vi "TestInsertIntoPanel_OK.vi"(8 "error in (no error)":errorcluster, 11 "TestCase in":refnum<class "TestProtectedSubpanel.lvclass">) -> (0 "error out":errorcluster, 3 "TestCase out":refnum<class "TestProtectedSubpanel.lvclass">)   [LabVIEW 2015, in "TestProtectedSubpanel.lvclass"]
uses:
  TestProtectedSubpanel.lvclass
  TestProtectedSubpanel.lvclass/TestProtectedSubpanel.ctl
  Framework/IViewable/ProtectedSubpanel/ProtectedSubpanel.lvclass
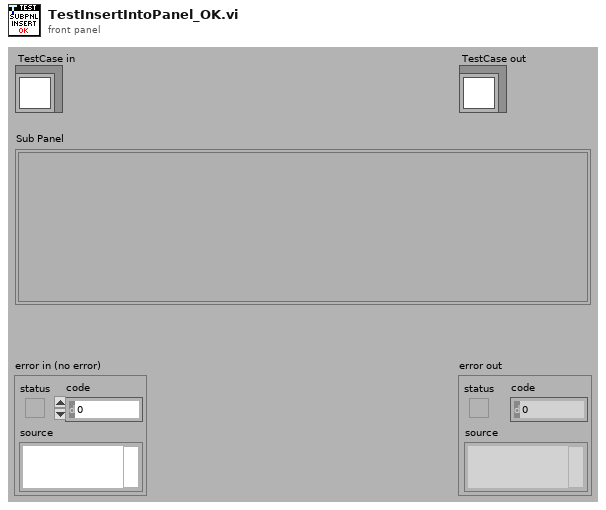
[diagram p1: front panel]
types:
  T1 = typedef "IViewable.lvlib/ProtectedSubpanel.lvclass/Protected Subpanel Reference.ctl" = refnum<data-value>
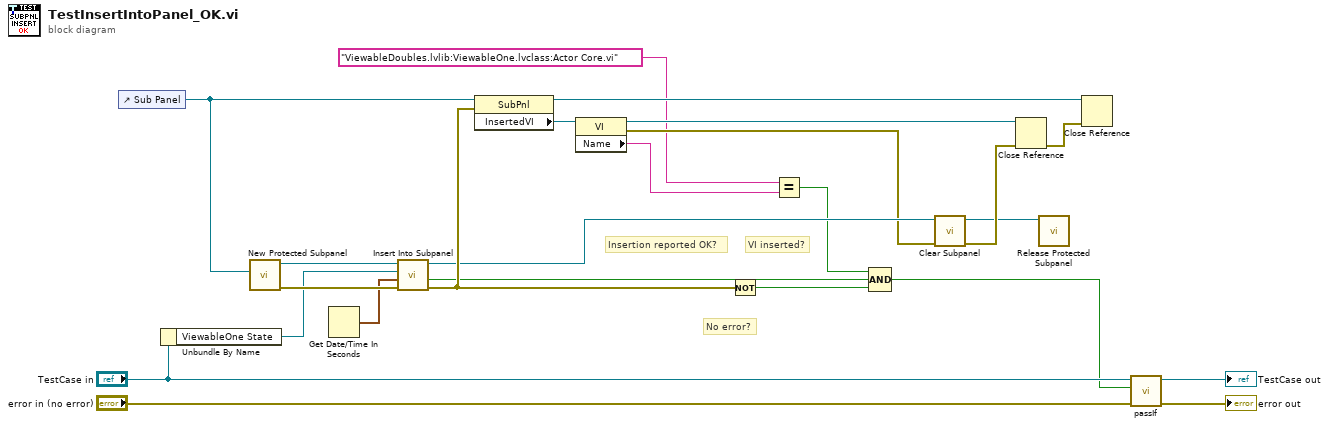
[diagram p0: block diagram]
diagram:
  # "Insertion reported OK?"
  # "No error?"
  # "VI inserted?"
  n1 = control-ref of="Sub Panel"() -> (w21:refnum<vi>)
  n2 = Unbundle By Name("TestCase in") -> ("ViewableOne State"=w5:refnum<class "IViewable.lvclass">)
  n3 = call "New Protected Subpanel.vi"("SubPnl Refnum"=w21) -> ("error out"=w12:errorcluster, "Protected Subpanel"=w20:T1)  [unwired: 9 in]
  n4 = Get Date/Time In Seconds() -> (seconds since 1Jan1904=w11:timestamp)
  n5 = call "Insert Into Subpanel.vi"("error in (no error)"=w12, "Insertion Request Time"=w11, "Viewable"=w5, "Protected Subpanel"=w20) -> ("error out"=w18:errorcluster, "Inserted?"=w10:bool, "Protected Subpanel"=w13:T1)  [unwired: 4 in, 1 out]
  n6 = property class="SubPnl"(reference=w21, error in=w18) -> (reference out=w15:refnum<vi>, "InsertedVI"=w17:refnum<vi>)  [unwired: 1 out]
  n7 = property class="VI"(reference=w17) -> (reference out=w7:refnum<vi>, error out=w4:errorcluster, "Name"=w16:string)  [unwired: 1 in]
  n8 = Not(x=w18) -> (.not. x?=w19:bool)
  n9 = Equal?(x="ViewableDoubles.lvlib:ViewableOne.lvclass:Actor Core.vi" ("y"), y=w16) -> (x = y?=w8:bool)
  n10 = Compound Arithmetic op=AND(w8, w10, w19) -> (w3:bool)
  n11 = call "Clear Subpanel.vi"("error in (no error)"=w4, "Protected Subpanel"=w13) -> ("error out"=w6:errorcluster, "Protected Subpanel Out"=w1:T1)  [unwired: 8 in]
  n12 = Close Reference(reference=w7, error in (no error)=w6) -> (error out=w14:errorcluster)
  n13 = call "Release Protected Subpanel.vi"("Protected Subpanel"=w1) -> ()  [unwired: 10 in, 1 out]
  n14 = Close Reference(reference=w15, error in (no error)=w14) -> ()  [unwired: 1 out]
  n15 = call-dynamic "passIf.vi"("error in (no error)"="error in (no error)", "pass"=w3, "TestCase in"="TestCase in") -> ("error out"=→"error out":errorcluster, "TestCase out"=→"TestCase out":refnum<class "TestProtectedSubpanel.lvclass">)  [unwired: 7 in]
